vi "testFilesPath.vi"(0 "reference in":refnum<class "Master Controller.lvclass">, 5 "error in (no error)":errorcluster) -> (14 "reference out":refnum<class "Master Controller.lvclass">, 19 "error out":errorcluster)   [LabVIEW 2016, in "Master Controller.lvclass"]
uses:
  Master Controller.lvclass
  File Controller_llb/File Controller.lvclass
  GUI/Project Panels_class/Project Panels.lvclass
  GUI/GUI Controller_llb/GUI Controller.lvclass
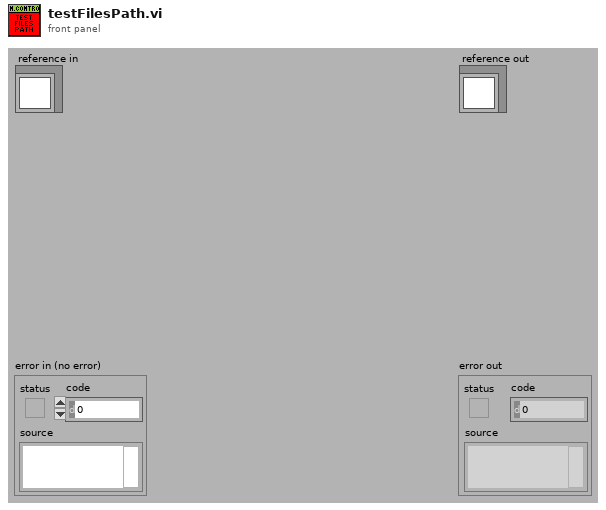
[diagram p1: front panel]
types:
  T1 = typedef "Master Controller.lvclass/ObjectAttributesRef.ctl" = refnum<data-value>
  T2 = typedef "Master Controller.lvclass/ObjectAttributes.ctl" = cluster{"MyAttribute":dbl, "Devices Controller_ref":refnum<class "Devices Controller.lvclass">, "File Controller_ref":refnum<class "File Controller.lvclass">, "Items Controller_ref":refnum<class "Items Controller.lvclass">, "GUI Controller_ref":refnum<class "GUI Controller.lvclass">, "NotificationController_ref":refnum<class "Notification Controller.lvclass">, "PartsTracking Controller_ref":refnum<class "PartsTracking Controller.lvclass">}
  T3 = cluster{"filePaths":path[], "outlookTemplatePaths":path[], "attachmentTemplatePaths":path[]}
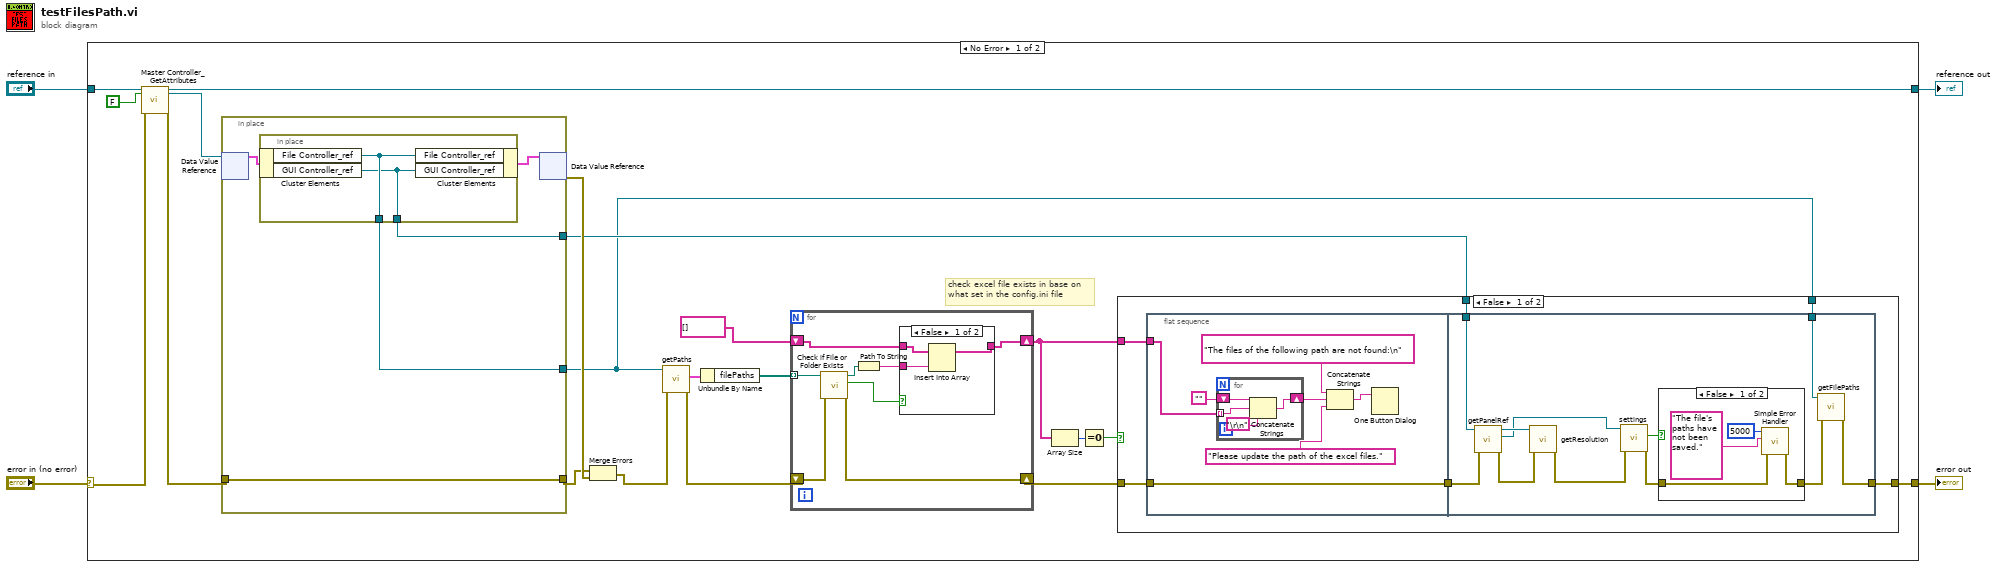
[diagram p0: block diagram]
diagram:
  n1 = case shown="No Error" "error in (no error)" {
    selector: "error in (no error)" -> [w20 w79]
    tunnel: [w9 w79] -> w3
    tunnel: [w18 w78] -> w1
    tunnel: "reference in" -> [w22 w78]
    frame No Error {
      # "check excel file exists in base on\nwhat set in the config.ini file"
      n2 = call "Master Controller_GetAttributes.vi"("reference in"=w22, "return data? (T)"=FALSE, "error in (no error)"=w20) -> ("reference out"=w18:refnum<class "Master Controller.lvclass">, "attributes ref"=w17:T1, "error out"=w19:errorcluster)  [unwired: 13 in, 1 out]
      n3 = in-place {
        in-place-border: w19 -> [w73]
        in-place-border: [w73] -> w23
        in-place-border: [w72] -> w5
        in-place-border: [w71] -> w11
        n4 = in-place-dvr #1(w17) -> (w74:T2)  [unwired: 1 out]
        n5 = in-place {
          in-place-border: [w77] -> w72
          in-place-border: [w76] -> w71
          n6 = in-place-cluster #2(w74) -> ("File Controller_ref"=w77:refnum<class "File Controller.lvclass">, "GUI Controller_ref"=w76:refnum<class "GUI Controller.lvclass">)
          n7 = in-place-cluster #2("File Controller_ref"=w77, "GUI Controller_ref"=w76) -> (w75:T2)
        }
        n8 = in-place-dvr #1(w75) -> (w24:errorcluster)  [unwired: 1 out]
      }
      n9 = Merge Errors(w23, w24) -> (w16:errorcluster)
      n10 = call "getPaths.vi"("error in (no error)"=w16, "reference in"=w5) -> ("error out"=w13:errorcluster, "paths"=w15:T3)  [unwired: 7 in, 1 out]
      n11 = Unbundle By Name(w15) -> ("filePaths"=w14:path[])
      n12 = for {
        tunnel: w14 -> [w66] mode=indexing
        shift-right: [w64] -> w10
        shift-left: w13 -> [w65]
        shift-right: [w60] -> w6
        shift-left: string[] [] -> [w63]
        n13 = call <vilib>:"Check if File or Folder Exists.vi"("error in (no error)"=w65, "path"=w66) -> ("error out"=w64:errorcluster, "file or folder exists?"=w59:bool, "dup path"=w62:path)  [unwired: 7 in]
        n14 = Path To String(path=w62) -> (string=w61:string)
        n15 = case shown="False" w59 {
          tunnel: w63 -> [w68 w70]
          tunnel: w61 -> [w69 _]
          tunnel: [w67 w70] -> w60
          frame False {
            n16 = Insert Into Array(array=w68, new element=w69) -> (w67:string[])  [unwired: 1 in]
          }
          frame True {
          }
        }
      }
      n17 = Array Size(array=w6) -> (size(s)=w8:i32)
      n18 = Equal To 0?(x=w8) -> (x = 0?=w7:bool)
      n19 = case shown="False" w7 {
        tunnel: w11 -> [w30 _]
        tunnel: w10 -> [w29 w58]
        tunnel: [w28 w58] -> w9
        tunnel: w6 -> [w26 _]
        tunnel: w5 -> [w25 _]
        frame False {
          n20 = flat-sequence {
            tunnel: w29 -> [w37]
            tunnel: [w37] -> w27
            tunnel: w26 -> [w31]
            tunnel: w30 -> [w52]
            tunnel: [w49] -> w28
            tunnel: w27 -> [w51]
            tunnel: w25 -> [w50]
            frame #0 {
              n21 = for {
                tunnel: w31 -> [w39] mode=indexing
                shift-right: [w41] -> w35
                shift-left: "" -> [w40]
                n22 = Concatenate Strings(w40, w39, "\r\n") -> (w41:string)
              }
              n23 = Concatenate Strings("The files of the following path are not found:\n", w35, "Please update the path of the excel files.") -> (w33:string)
              n24 = One Button Dialog(message=w33) -> ()  [unwired: 1 in, 1 out]
            }
            frame #1 {
              n25 = call "getPanelRef.vi"("error in (no error)"=w51, "reference in"=w52) -> ("error out"=w47:errorcluster, "project_panels_ref"=w45:refnum<class "Project Panels.lvclass">, "reference out"=w48:refnum<class "GUI Controller.lvclass">)  [unwired: 7 in]
              n26 = call "getResolution.vi"("reference in"=w48, "error in (no error)"=w47) -> ("error out"=w46:errorcluster)  [unwired: 6 in, 2 out]
              n27 = call "settings.vi"("error in (no error)"=w46, "reference in"=w45) -> ("error out"=w44:errorcluster, "Saved?"=w42:bool)  [unwired: 7 in, 1 out]
              n28 = case shown="False" w42 {
                tunnel: w44 -> [w56 w57]
                tunnel: [w55 w57] -> w43
                frame False {
                  n29 = call <vilib>:"Simple Error Handler.vi"("error code (no error:0)"=5000, "error source (\" \")"="The file's paths have not been saved." ("error source (\" \")"), "error in (no error)"=w56) -> ("error out"=w55:errorcluster)  [unwired: 2 in, 4 out]
                }
                frame True {
                }
              }
              n30 = call "getFilePaths.vi"("error in (no error)"=w43, "reference in"=w50) -> ("error out"=w49:errorcluster)  [unwired: 8 in, 1 out]
            }
          }
        }
        frame True {
        }
      }
    }
    frame Error {
    }
  }
  "error out" <- w3
  "reference out" <- w1
